vi "TEST.vi"() -> ()   [LabVIEW 2010]
uses:
  D:/PROJECT/Inteliss/pc_test_app/Canopen_project/canopenlib_cli.dll
  pc_test_app/Canopen_project/canopenlib_cli.dll
  CANOpen.lvlib
panel:
  out "canHardwareConnect":i32(ring) items=["CANOPEN_OK"=0, "CANOPEN_ERROR"=-255, "CANOPEN_ERROR_ASYNC_TRANSFER_ENABLED"=-114, "CANOPEN_ASYNC_TRANSFER"=-113, "CANOPEN_ERROR_NOT_EDS_DCF_CONFIGURED"=-112, "CANOPEN_ERROR_FILE_NOT_FOUND"=-111, "CANOPEN_ERROR_NOT_IMPLEMENTED"=-110, "CANOPEN_ERROR_NO_MESSAGE"=-109, "CANOPEN_UNSUPPORTED_BITRATE"=-108, "CANOPEN_OUT_OF_CAN_INTERFACES"=-107, "CANOPEN_ERROR_DRIVER"=-106, "CANOPEN_ERROR_HW_UNDEFINED"=-105, "CANOPEN_ERROR_HW_NOT_CONNECTED"=-104, "CANOPEN_ERROR_HW_CONNECTED"=-103, "CANOPEN_ERROR_CAN_LAYER_OVRFLOW"=-102, "CANOPEN_ERROR_CAN_LAYER"=-101, "CANOPEN_CAN_LAYER_FAILED"=-100, "CANOPEN_NODE_ID_OUT_OF_RANGE"=-15, "CANOPEN_INTERNAL_STATE_ERROR"=-14, "CANOPEN_CMD_SPEC_UNKNOWN_OR_INVALLD"=-13, "CANOPEN_ERR_DEFINED_BY_APPL"=-12, "CANOPEN_OUT_OF_MEM"=-11, "CANOPEN_REMOTE_NODE_ABORT"=-10, "CANOPEN_APP_BUF_OUT_OF_RANGE"=-9, "CANOPEN_OBJECT_MISSMATCH"=-8, "CANOPEN_BUFFER_TOO_SMALL"=-7, "CANOPEN_TOGGLE"=-6, "CANOPEN_MSG_NOT_PROCESSED"=-5, "CANOPEN_TIMEOUT"=-4, "CANOPEN_UNEXPECTED_CCS"=-3, "CANOPEN_UNEXPECTED_SCS"=-2, "CANOPEN_ARG_ERROR"=-1]
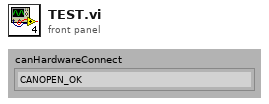
[diagram p1: front panel]
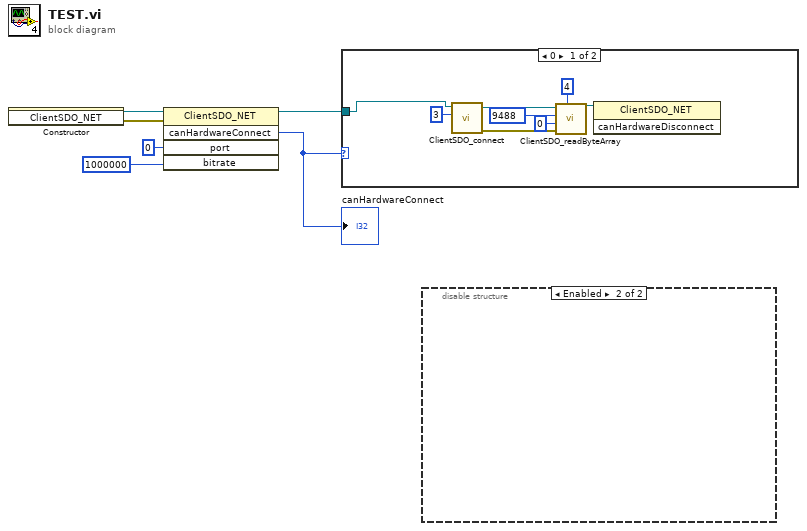
[diagram p0: block diagram]
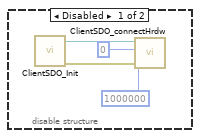
[diagram p3: hidden frame]
diagram:
  n1 = constructor class="ClientSDO_NET"() -> (reference out=w5:refnum<k24>, error out=w6:errorcluster)  [unwired: 3 in, 1 out]
  n2 = invoke class="ClientSDO_NET" method="canHardwareConnect"(reference=w5, error in=w6, "port"=0, "bitrate"=1000000) -> (reference out=w1:refnum<k24>, "canHardwareConnect"=w2:i32)  [unwired: 1 in, 3 out]
  "canHardwareConnect" <- w2
  n3 = case shown="0" w2 {
    tunnel: w1 -> [w7 _]
    frame 0 {
      n4 = call "ClientSDO_connect.vi"("node_id"=u8 3, "ClientSDO Ref in"=w7) -> ("error out"=w12:errorcluster, "ClientSDO Ref out"=w13:refnum<k24>)  [unwired: 7 in, 1 out]
      n5 = call "ClientSDO_readByteArray.vi"("length"=4, "error in (no error)"=w12, "sub_index"=u8 0, "object_index"=u16 9488, "ClientSDO Ref in"=w13) -> ("ClientSDO Ref out"=w8:refnum<k24>)  [unwired: 2 in, 4 out]
      n6 = invoke class="ClientSDO_NET" method="canHardwareDisconnect"(reference=w8) -> ()  [unwired: 2 in, 3 out]
    }
    frame 1, Default {
    }
  }
  n7 = disable-structure shown="Enabled" {
    frame Disabled {
      n8 = call "ClientSDO_Init.vi"() -> ("error out"=w17:errorcluster, "ClientSDO Ref out"=w18:refnum<k24>)  [unwired: 10 in]
      n9 = call "ClientSDO_connectHrdw.vi"("error in (no error)"=w17, "bitrate"=1000000, "port"=0, "ClientSDO Ref in"=w18) -> ()  [unwired: 5 in, 3 out]
    }
    frame Enabled {
    }
  }
